vi "RF Power On-Off.vi"(8 "error in (no error)":errorcluster, 9 "RF Power State (T: On)":bool, 11 "N5222A PNA in":refnum<class "N5222A PNA.lvclass">) -> (0 "error out":errorcluster, 3 "N5222A PNA out":refnum<class "N5222A PNA.lvclass">)   [LabVIEW 2019, in "N5222A PNA.lvclass"]
doc: "turn output off when repatching the cables"
uses:
  N5222A PNA.lvclass
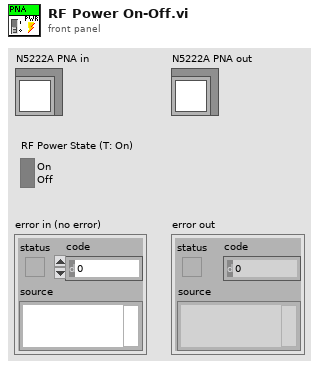
[diagram p1: front panel]
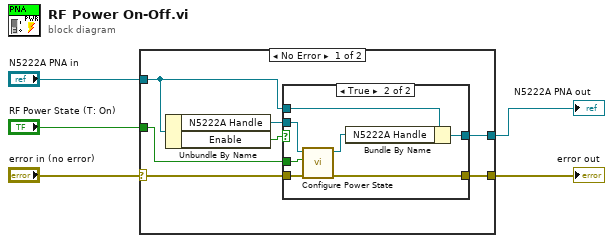
[diagram p0: block diagram]
diagram:
  n1 = case shown="No Error" "error in (no error)" {
    selector: "error in (no error)" -> [w8 w23]
    tunnel: [w7 w23] -> w4
    tunnel: [w10 w22] -> w2
    tunnel: "N5222A PNA in" -> [w11 w22]
    tunnel: "RF Power State (T: On)" -> [w12 _]
    frame No Error {
      n2 = Unbundle By Name(w11) -> ("N5222A Handle"=w9:refnum<visa-resource-name>, "Enable"=w6:bool)
      n3 = case shown="True" w6 {
        tunnel: w12 -> [_ w21]
        tunnel: w11 -> [w14 w20]
        tunnel: [w14 w19] -> w10
        tunnel: w9 -> [_ w18]
        tunnel: w8 -> [w13 w16]
        tunnel: [w13 w15] -> w7
        frame False {
        }
        frame True {
          n4 = call <instrlib>:"Configure Power State.vi"("Error In (no error)"=w16, "RF Power State (T: On)"=w21, "VISA Resource Name"=w18) -> ("Error Out"=w15:errorcluster, "VISA Resource Name Out"=w17:refnum<visa-resource-name>)  [unwired: 7 in]
          n5 = Bundle By Name(cluster=w20, "N5222A Handle"=w17) -> (w19:refnum<class "N5222A PNA.lvclass">)
        }
      }
    }
    frame Error {
    }
  }
  "error out" <- w4
  "N5222A PNA out" <- w2
